vi "Save Grouped Tags To Disk.vi"(7 "Force Lookup? (F)":bool, 8 "error in (no error)":errorcluster, 10 "Group":string, 11 "XML File Path":path) -> (0 "error out":errorcluster)   [LabVIEW 2020, in "Current Value Table(Rebuild).lvlib"]
doc: "This VI will save a single group from the CVT to disk. On the first call, it will produce a list of every tag in the CVT, and fetch the lookup information for each tag. Then, it will retrieve the actual data and format it into a list of tags and save those tags to disk at the path specified. On subsequent calls, unless the (Re)initialize? boolean is set, it will simply store those same tags to disk even if more tags have been added. \nNOTE: The VIs called by this function are reentrant, so each instance of this top level VI will retain its own set of tags. This allows for multiple groups to be saved, but may cause confusing behavior."
uses:
  Current Value Table(Rebuild).lvlib
  <vilib>/Utility/xml.llb/Write to XML File(string).vi
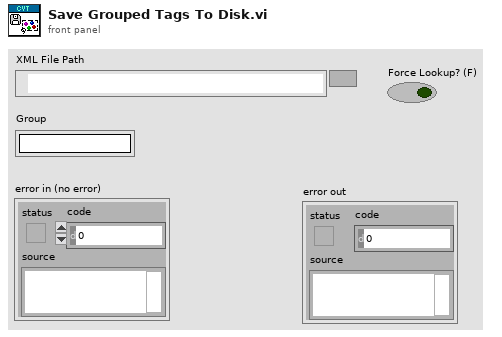
[diagram p1: front panel]
types:
  T1 = typedef "Current Value Table(Rebuild).lvlib/File Format.ctl" = cluster{"Tags":T2[], "Group Listings":T4[]}
  T2 = typedef "Current Value Table(Rebuild).lvlib/Single Tag.ctl" = cluster{"Data Type":T3, "Name":string, "Value":string, "Description":string}
  T3 = typedef "Current Value Table(Rebuild).lvlib/Data Types.ctl" = enum16{"Double", "Single", "I64", "I32", "I16", "I8", "U64", "U32", "U16", "U8", "String", "Boolean", "Array of U8", "Array of U16", "Array of U32", "Array of U64", "Array of I64", "Array of I32", "Array of I16", "Array of I8", "Array of Double", "Array of Single", "Array of Boolean", "Array of String"}
  T4 = typedef "Current Value Table(Rebuild).lvlib/Tag Grouping set.ctl" = cluster{"Group":string, "Tag Names":string[]}
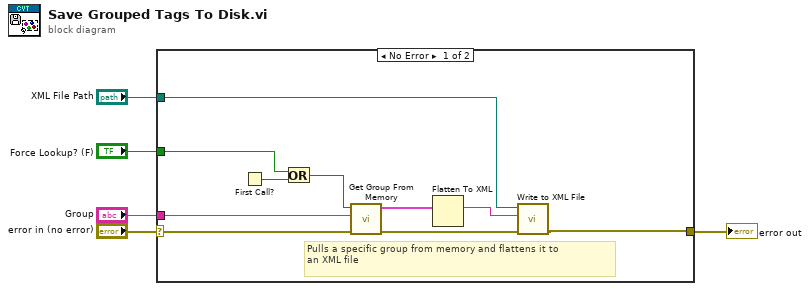
[diagram p0: block diagram]
diagram:
  n1 = case shown="No Error" "error in (no error)" {
    selector: "error in (no error)" -> [w15 w16]
    tunnel: "XML File Path" -> [w9 _]
    tunnel: [w8 w16] -> w3
    tunnel: "Group" -> [w12 _]
    tunnel: "Force Lookup? (F)" -> [w6 _]
    frame No Error {
      # "Pulls a specific group from memory and flattens it to\nan XML file"
      n2 = First Call?() -> (First Call?: T/F=w13:bool)
      n3 = Or(x=w6, y=w13) -> (x .or. y?=w14:bool)
      n4 = call "Get Group From Memory.vi"("error in (no error)"=w15, "Group"=w12, "(Re)initialize? (F)"=w14) -> ("error out"=w10:errorcluster, "CVT File Data"=w11:T1)  [unwired: 7 in]
      n5 = Flatten To XML(6:w11) -> (2:w7:string)
      n6 = call-poly <vilib>:"Write to XML File.vi"("error in (no error)"=w10, "XML Input"=w7, "XML File Path"=w9) -> ("error out"=w8:errorcluster)  [unwired: 6 in, 2 out]
    }
    frame Error {
    }
  }
  "error out" <- w3
